vi "Start Game.vi"(8 "error in (no error)":errorcluster, 9 "Replication Rounds":u32=50, 10 "Board Size":i32=150, 11 "Game in":refnum<class "Game.lvclass">) -> (0 "error out":errorcluster, 3 "Game out":refnum<class "Game.lvclass">)   [LabVIEW 2020, in "SquareBattle.lvlib" / "Game.lvclass"]
uses:
  Game.lvclass
  Game.lvclass/Game.ctl
  Team/Team.lvclass
  Map/Map.lvclass
  Square/Square.lvclass
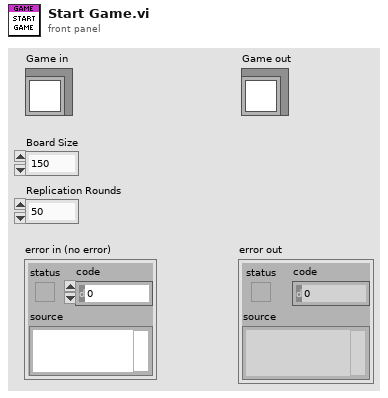
[diagram p1: front panel]
types:
  T1 = typedef "SquareBattle.lvlib/Position.ctl" = cluster{"Row":i32, "Col":i32}
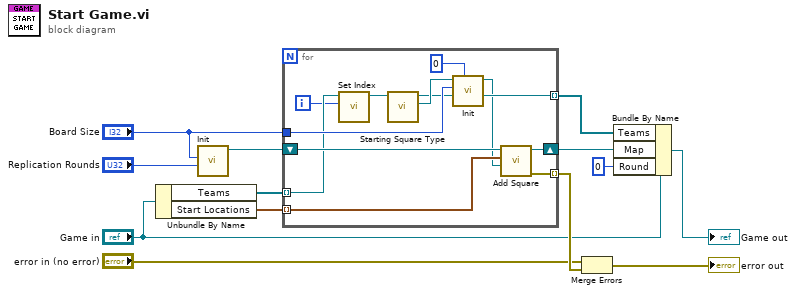
[diagram p0: block diagram]
diagram:
  n1 = Unbundle By Name("Game in") -> ("Teams"=w2:refnum<class "Team.lvclass">[], "Start Locations"=w1:T1[])
  n2 = call "Init.vi"("Replication Rounds"="Replication Rounds", "Size"="Board Size") -> ("Map out"=w11:refnum<class "Map.lvclass">)  [unwired: 8 in, 1 out]
  n3 = for {
    shift-right: [w25] -> w9
    shift-left: w11 -> [w26]
    tunnel: "Board Size" -> [w21]
    tunnel: [w22] -> w7 mode=indexing
    tunnel: [w24] -> w13 mode=indexing
    tunnel: w2 -> [w15] mode=indexing
    tunnel: w1 -> [w20] mode=indexing
    i -> [w14]
    n4 = call "Set Index.vi"("Index"=w14, "Team in"=w15) -> ("Team out"=w16:refnum<class "Team.lvclass">)  [unwired: 9 in]
    n5 = call-dynamic "Starting Square Type.vi"("Team in"=w16) -> ("Square"=w19:refnum<class "Square.lvclass">, "Team out"=w18:refnum<class "Team.lvclass">)  [unwired: 9 in]
    n6 = call "Init.vi"("Round"=u32 0, "Team in"=w18, "Board Size"=w21, "Square in"=w19) -> ("Team out"=w22:refnum<class "Team.lvclass">, "Square out"=w17:refnum<class "Square.lvclass">)  [unwired: 6 in]
    n7 = call "Add Square.vi"("Square"=w17, "Position"=w20, "Map in"=w26) -> ("error out"=w24:errorcluster, "Map out"=w25:refnum<class "Map.lvclass">)  [unwired: 7 in]
  }
  n8 = Merge Errors("error in (no error)", w13) -> (→"error out":errorcluster)
  n9 = Bundle By Name(cluster="Game in", "Teams"=w7, "Map"=w9, "Round"=u32 0) -> (→"Game out":refnum<class "Game.lvclass">)
